vi "Get Tag Content.vi"(10 "Tag":string="[~<>]*", 11 "xml string in":string) -> (1 "Tag with Content":string, 2 "Tag content":string, 3 "After end of tag":string)   [LabVIEW 2020, in "Comparator.lvclass"]
uses:
  Comparator.lvclass
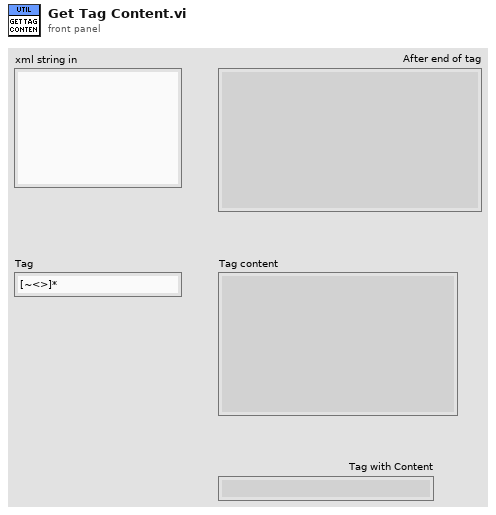
[diagram p1: front panel]
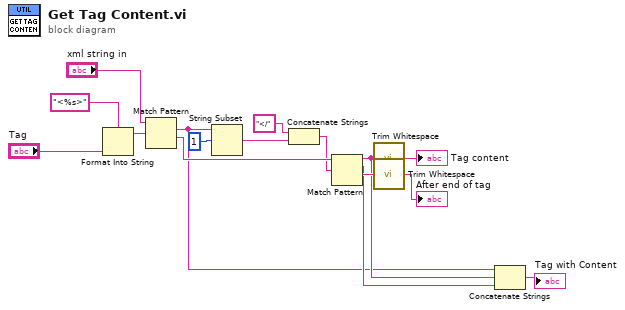
[diagram p0: block diagram]
diagram:
  n1 = Format Into String(format string="<%s>", "Tag") -> (resulting string=w16:string)  [unwired: 2 in, 1 out]
  n2 = Match Pattern(string="xml string in", regular expression=w16) -> (match substring=w1:string, after substring=w14:string)  [unwired: 1 in, 2 out]
  n3 = String Subset(string=w1, offset (0)=1) -> (substring=w6:string)  [unwired: 1 in]
  n4 = Concatenate Strings("</" ("substring (\"\")"), w6) -> (w11:string)
  n5 = Match Pattern(string=w14, regular expression=w11) -> (before substring=w4:string, match substring=w3:string, after substring=w12:string)  [unwired: 1 in, 1 out]
  n6 = call <vilib>:"Trim Whitespace.vi"("string"=w4) -> ("trimmed string"=→"Tag content":string)  [unwired: 1 in]
  n7 = call <vilib>:"Trim Whitespace.vi"("string"=w12) -> ("trimmed string"=→"After end of tag":string)  [unwired: 1 in]
  n8 = Concatenate Strings(w1, w4, w3) -> (→"Tag with Content":string)
